vi "get waveform - voltage range scaled.vi"(8 "error in (no error)":errorcluster caption="에러 입력(에러 없음)", 11 "WAV File 입력":refnum<class "WAV File.lvclass">) -> (0 "error out":errorcluster caption="에러 출력", 2 "scaled waveform":waveform(dbl), 3 "WAV File 출력":refnum<class "WAV File.lvclass">)   [LabVIEW 2020, in "WAV File.lvclass"]
uses:
  WAV File.lvclass
  WAV File.lvclass/WAV File.ctl
  Waveform Obj/Waveform Obj.lvclass/Waveform Obj.ctl
  Accessors/Read sound format.vi
  Waveform Obj/Accessors/Read voltage range.vi
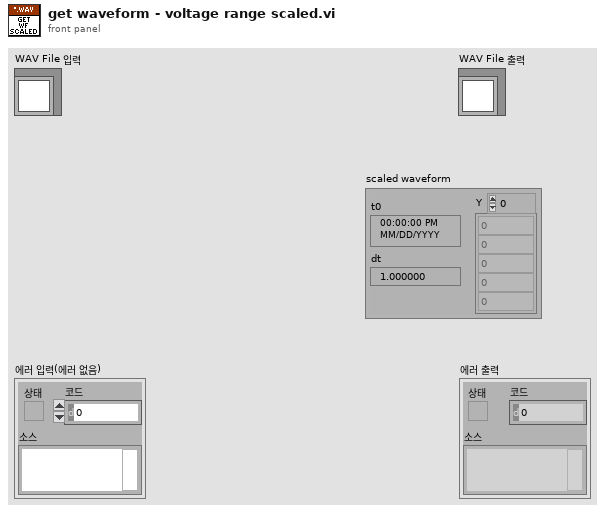
[diagram p1: front panel]
types:
  T1 = typedef "Sound Data Format.ctl" = cluster{"sample rate (S/s)":dbl, "number of channels":i32, "bits per sample":i32}
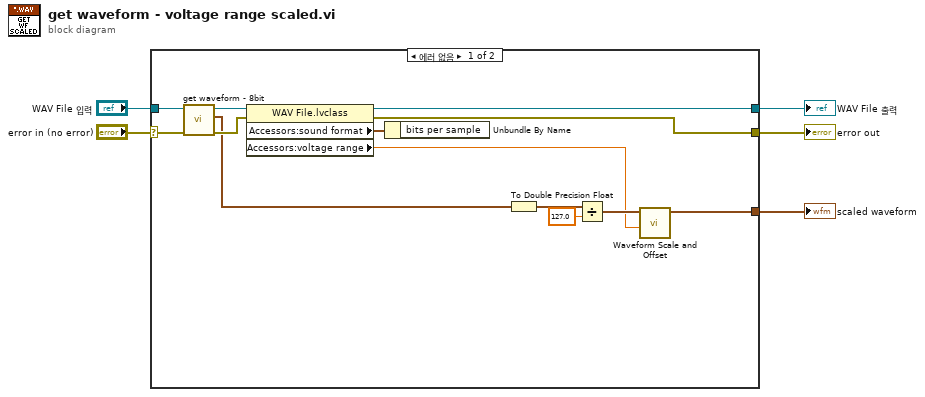
[diagram p0: block diagram]
diagram:
  n1 = case shown="에러 없음" "error in (no error)" {
    selector: "error in (no error)" -> [w18 w20]
    tunnel: [w13 w20] -> w5
    tunnel: [w12 w19] -> w3
    tunnel: "WAV File 입력" -> [w9 w19]
    tunnel: [w14 _] -> w4
    frame No Error {
      n2 = call-dynamic "get waveform - 8bit.vi"("error in (no error)"=w18, "WAV File 입력"=w9) -> ("error out"=w10:errorcluster, "8bit waveform"=w7:waveform(i8), "WAV File 출력"=w8:refnum<class "WAV File.lvclass">)  [unwired: 6 in, 1 out]
      n3 = property class="WAV File.lvclass"(reference=w8, error in=w10) -> (reference out=w12:refnum<class "WAV File.lvclass">, error out=w13:errorcluster, "Accessors:sound format"=w6:T1, "Accessors:voltage range"=w11:dbl)
      n4 = Unbundle By Name(w6) -> ()  [unwired: 1 out]
      n5 = To Double Precision Float(number=w7) -> (double precision float=w17:waveform(dbl))
      n6 = Divide(x=w17, y=127.0) -> (x/y=w15:waveform(dbl))
      n7 = call <vilib>:"Waveform Scale and Offset.vi"("scale"=w11, "waveform in"=w15) -> ("waveform out"=w14:waveform(dbl))  [unwired: 8 in, 1 out]
    }
    frame Error {
    }
  }
  "error out" <- w5
  "WAV File 출력" <- w3
  "scaled waveform" <- w4
